vi "FLC_Temperature_Sederhana.vi"() -> ()   [LabVIEW 2020]
uses:
  <vilib>/Instr/_visa.llb/VISA Configure Serial Port (Instr).vi
  <vilib>/addons/Fuzzy Logic/FL Fuzzy Controller (MISO).vi
  <vilib>/addons/Fuzzy Logic/NI_Fuzzy_Logic_API.lvlib
panel:
  out "Control Value (CV) - PWM":dbl(knob) scale=0.0..255.0
  out "Rule":picture
  out "Membership CV":picture
  out "Membership Error":picture
  out "Membership Temperature":picture
  out "Control Value (CV)":dbl(slide) scale=0.0..100.0
  out "Error":i32(slide) scale=-30.0..30.0
  out "Temperature Aktual (PV)":i32(slide) scale=0.0..45.0
  in  "stop":bool
  in  "Set Point (SP)":i32(slide) scale=0.0..50.0
  in  "baud rate (9600)":u32=9600
  in  "VISA resource name":refnum<visa-resource-name>
  # "OUTPUT"
  # "INPUT"
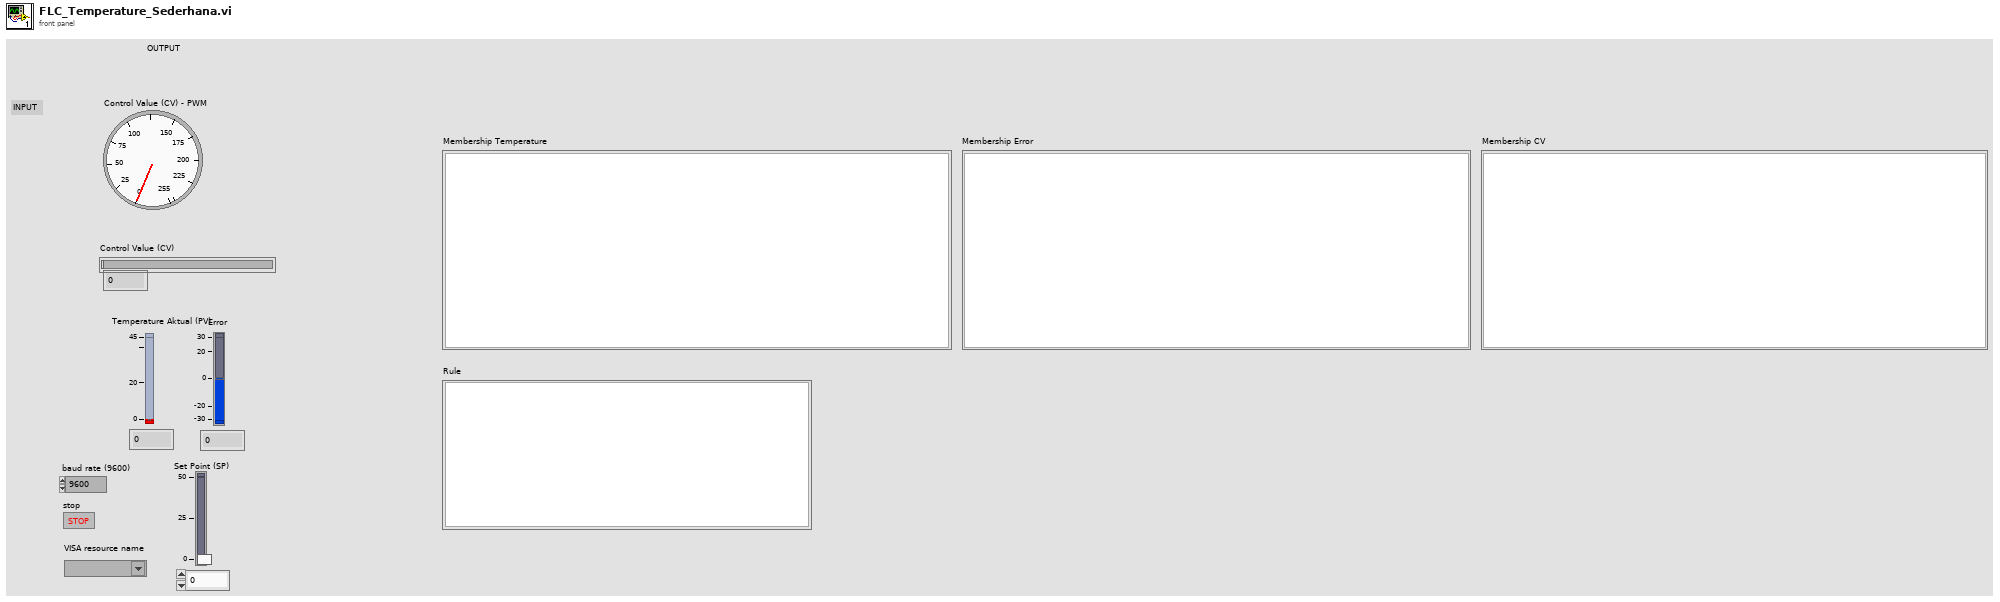
[diagram p1: front panel]
types:
  T1 = typedef "imagedata.ctl" = cluster{"image type":i32, "image depth":i32, "image":u8[], "mask":u8[], "colors":u32[], "Rectangle":cluster{"left":i16, "top":i16, "right":i16, "bottom":i16}}
  T2 = typedef "NI_Fuzzy_Logic_API.lvlib/FL System.ctl" = cluster{"input variables":T3[], "output variables":T3[], "rules":T6[], "defuzzification method":T12, "description":string, "user MF interpolating polynomials":T13[]}
  T3 = typedef "NI_Fuzzy_Logic_API.lvlib/FL Variable.ctl" = cluster{"name":string, "range":dbl[], "MFs":T4[]}
  T4 = typedef "NI_Fuzzy_Logic_API.lvlib/FL Membership Function.ctl" = cluster{"name":string, "shape":T5, "points":dbl[], "color":u32, "user-defined shape index":i32}
  T5 = typedef "NI_Fuzzy_Logic_API.lvlib/FL Membership Function Shape.ctl" = u16
  T6 = typedef "NI_Fuzzy_Logic_API.lvlib/FL Rule.ctl" = cluster{"antecedents":T7[], "antecedent connective":T9, "consequents":T10[], "consequent implication":T11, "degree of support":dbl}
  T7 = typedef "NI_Fuzzy_Logic_API.lvlib/FL Antecedent.ctl" = cluster{"Var Index":i32, "MF Index":i32, "Cond":T8}
  T8 = typedef "NI_Fuzzy_Logic_API.lvlib/FL Modifier.ctl" = u16
  T9 = typedef "NI_Fuzzy_Logic_API.lvlib/FL Antecedent Connective.ctl" = u16
  T10 = typedef "NI_Fuzzy_Logic_API.lvlib/FL Consequent.ctl" = cluster{"Var Index":i32, "MF Index":i32, "Cond":T8}
  T11 = typedef "NI_Fuzzy_Logic_API.lvlib/FL Consequent Implication.ctl" = u16
  T12 = typedef "NI_Fuzzy_Logic_API.lvlib/FL Defuzzification.ctl" = u16
  T13 = typedef "NI_Fuzzy_Logic_API.lvlib/FL Interpolating polynomials.ctl" = cluster{"X":dbl[], "Y":dbl[], "Y(x) coeff":dbl[][], "X(y) coeff":dbl[][], "Area(y) coeff":dbl[][], "coa_x(y) coeff":dbl[][]}
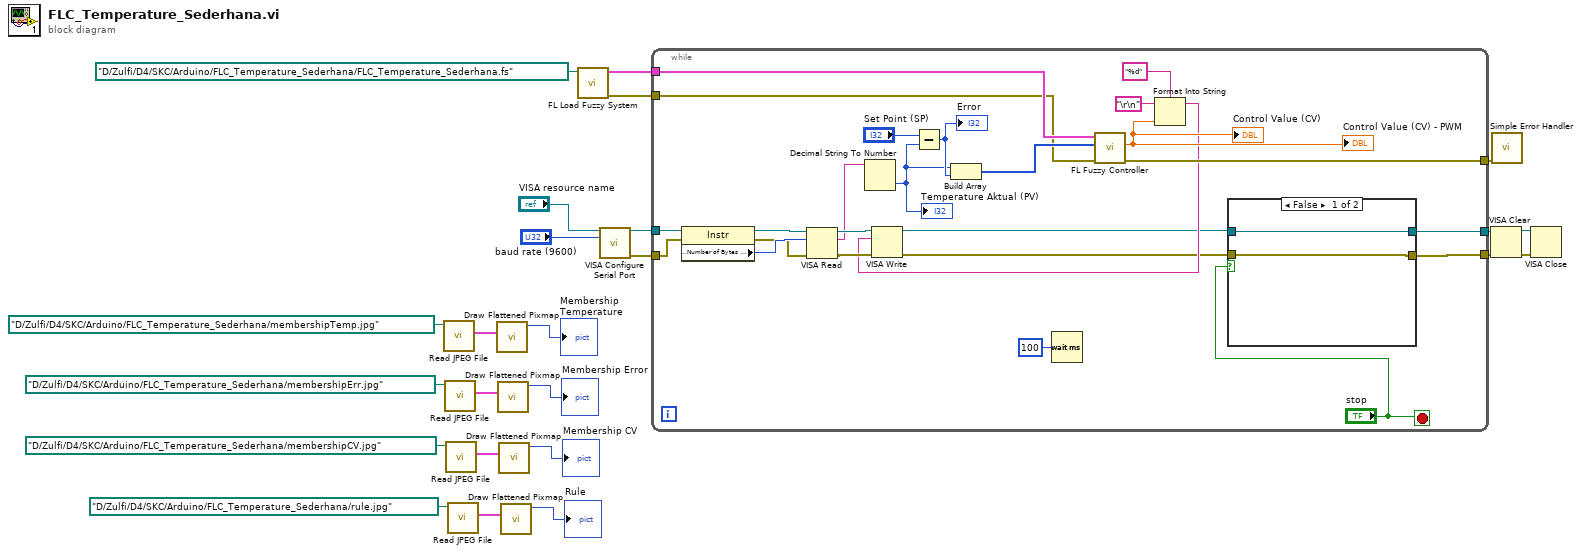
[diagram p0: block diagram]
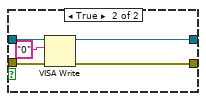
[diagram p2: hidden frame]
diagram:
  n1 = call <vilib>:"Read JPEG File.vi"("path to JPEG file"=path "D:/Zulfi/D4/SKC/Arduino/FLC_Temperature_Sederhana/membershipTemp.jpg") -> ("image data"=w12:T1)  [unwired: 8 in, 2 out]
  n2 = call <vilib>:"Read JPEG File.vi"("path to JPEG file"=path "D:/Zulfi/D4/SKC/Arduino/FLC_Temperature_Sederhana/membershipErr.jpg") -> ("image data"=w10:T1)  [unwired: 8 in, 2 out]
  n3 = call <vilib>:"Read JPEG File.vi"("path to JPEG file"=path "D:/Zulfi/D4/SKC/Arduino/FLC_Temperature_Sederhana/membershipCV.jpg") -> ("image data"=w8:T1)  [unwired: 8 in, 2 out]
  n4 = call <vilib>:"Read JPEG File.vi"("path to JPEG file"=path "D:/Zulfi/D4/SKC/Arduino/FLC_Temperature_Sederhana/rule.jpg") -> ("image data"=w6:T1)  [unwired: 8 in, 2 out]
  n5 = call <vilib>:"Draw Flattened Pixmap.vi"("image data"=w12) -> ("new picture"=→"Membership Temperature":picture)  [unwired: 8 in]
  n6 = call <vilib>:"Draw Flattened Pixmap.vi"("image data"=w10) -> ("new picture"=→"Membership Error":picture)  [unwired: 8 in]
  n7 = call <vilib>:"Draw Flattened Pixmap.vi"("image data"=w8) -> ("new picture"=→"Membership CV":picture)  [unwired: 8 in]
  n8 = call <vilib>:"Draw Flattened Pixmap.vi"("image data"=w6) -> ("new picture"=→"Rule":picture)  [unwired: 8 in]
  n9 = call <vilib>:"FL Load Fuzzy System.vi"("file path"=path "D:/Zulfi/D4/SKC/Arduino/FLC_Temperature_Sederhana/FLC_Temperature_Sederhana.fs") -> ("error out"=w19:errorcluster, "fuzzy system out"=w20:T2)  [unwired: 9 in]
  n10 = call-poly "VISA Configure Serial Port"("VISA resource name"="VISA resource name", "baud rate (9600)"="baud rate (9600)") -> ("VISA resource name out"=w24:refnum<visa-resource-name>, "error out"=w23:errorcluster)  [unwired: 12 in]
  n11 = while {
    tunnel: w24 -> [w49]
    tunnel: w23 -> [w48]
    tunnel: w20 -> [w38]
    tunnel: w19 -> [w37]
    tunnel: [w36] -> w18
    tunnel: [w29] -> w15
    tunnel: [w27] -> w14
    stop <- "stop" stop-if-true
    n12 = property class="Instr"(reference=w49, error in=w48) -> (reference out=w47:refnum<visa-resource-name>, error out=w45:errorcluster, "Serial Settings:Number of Bytes at Serial Port"=w46:u32)
    n13 = VISA Read(VISA resource name=w47, byte count=w46, error in (no error)=w45) -> (VISA resource name out=w44:refnum<visa-resource-name>, read buffer=w42:string, error out=w43:errorcluster)  [unwired: 1 out]
    n14 = Decimal String To Number(string=w42) -> (number=w25:i32)  [unwired: 2 in, 1 out]
    "Temperature Aktual (PV)" <- w25
    n15 = Subtract(x="Set Point (SP)", y=w25) -> (x-y=w39:i32)
    "Error" <- w39
    n16 = Build Array(w25, w39) -> (w40:i32[])
    n17 = Wait (ms)(milliseconds to wait=u32 100) -> ()  [unwired: 1 out]
    n18 = call-poly <vilib>:"FL Fuzzy Controller.vi"("error in (no error)"=w37, "input values"=w40, "fuzzy system in"=w38) -> ("error out"=w36:errorcluster, "output value"=w35:dbl)  [unwired: 4 in, 3 out]
    "Control Value (CV)" <- w35
    "Control Value (CV) - PWM" <- w35
    n19 = Format Into String(format string="%d", initial string="\r\n", w35) -> (resulting string=w33:string)  [unwired: 1 in, 1 out]
    n20 = VISA Write(VISA resource name=w44, write buffer=w33, error in (no error)=w43) -> (VISA resource name out=w32:refnum<visa-resource-name>, error out=w28:errorcluster)  [unwired: 1 out]
    n21 = case shown="False" "stop" {
      tunnel: w32 -> [w51 w56]
      tunnel: w28 -> [w50 w53]
      tunnel: [w51 w54] -> w29
      tunnel: [w50 w52] -> w27
      frame False {
      }
      frame True {
        n22 = VISA Write(VISA resource name=w56, write buffer="0", error in (no error)=w53) -> (VISA resource name out=w54:refnum<visa-resource-name>, error out=w52:errorcluster)  [unwired: 1 out]
      }
    }
  }
  n23 = VISA Clear(VISA resource name=w15, error in (no error)=w14) -> (VISA resource name out=w17:refnum<visa-resource-name>, error out=w16:errorcluster)
  n24 = call <vilib>:"Simple Error Handler.vi"("error in (no error)"=w18) -> ()  [unwired: 4 in, 5 out]
  n25 = VISA Close(VISA resource name=w17, error in (no error)=w16) -> ()  [unwired: 1 out]
